vi "PathPlanning-int.vi"(0 "Map&Nodes":T1, 1 "error in (no error)":errorcluster) -> (2 "Path":i32[](array[numeric]), 3 "Coordinates":cluster{"X":dbl, "Y":dbl}[](array[cluster]), 4 "error out":errorcluster)   [LabVIEW 2009]
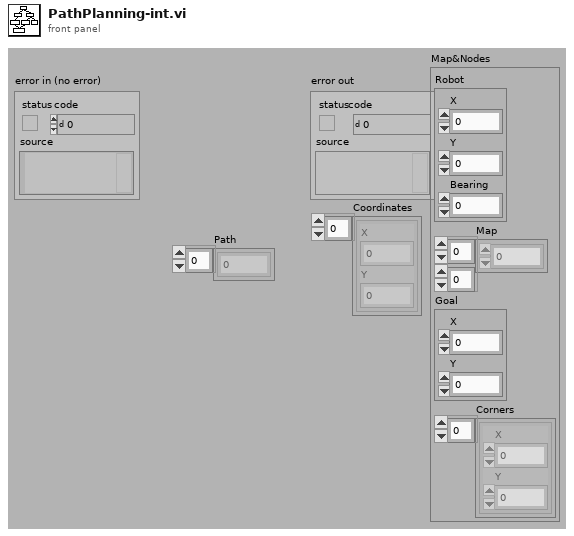
[diagram p1: front panel]
types:
  T1 = cluster{"Robot":cluster{"X":i16, "Y":i16, "Bearing":dbl}, "Map":i8[][], "Goal":cluster{"X":i16, "Y":i16}, "Corners":cluster{"X":i16, "Y":i16}[]}
  T2 = cluster{"From node":cluster{"X":i16, "Y":i16}, "Dest node":cluster{"X":i16, "Y":i16}, "Distance":dbl, "Dest node no":i32, "From node no":i32}[]
  T3 = cluster{"From node":cluster{"X":i16, "Y":i16}, "Dest node":cluster{"X":i16, "Y":i16}, "Distance":dbl, "Dest node no":i32, "From node no":i32}
  T4 = cluster{"From node":cluster{"X":dbl, "Y":dbl}, "Dest node":cluster{"X":dbl, "Y":dbl}, "Distance":dbl, "Dest node no":i32, "From node no":i32}
  T5 = cluster{"From node":cluster{"X":dbl, "Y":dbl}, "Dest node":cluster{"X":dbl, "Y":dbl}, "Distance":dbl, "Dest node no":i32, "From node no":i32}[]
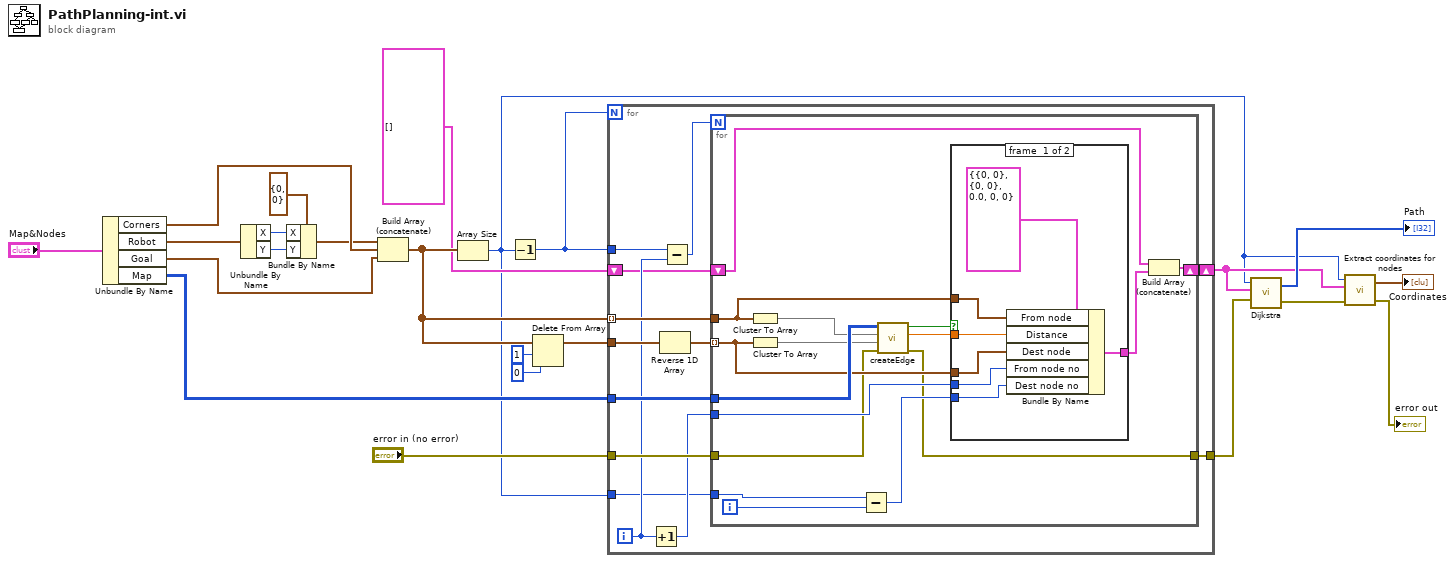
[diagram p0: block diagram]
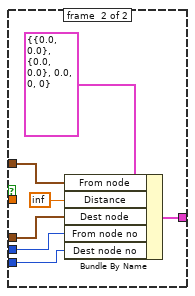
[diagram p2: hidden frame]
diagram:
  n1 = Unbundle By Name("Map&Nodes") -> ("Corners"=w15:cluster{"X":i16, "Y":i16}[], "Robot"=w19:cluster{"X":i16, "Y":i16, "Bearing":dbl}, "Goal"=w14:cluster{"X":i16, "Y":i16}, "Map"=w20:i8[][])
  n2 = Unbundle By Name(w19) -> ("X"=w18:i16, "Y"=w17:i16)
  n3 = Bundle By Name(cluster=cluster{"X":i16, "Y":i16} {"X"=0, "Y"=0} ("Robot 2"), "X"=w18, "Y"=w17) -> (w13:cluster{"X":i16, "Y":i16})
  n4 = Build Array (concatenate)(w13, w15, w14) -> (w12:cluster{"X":i16, "Y":i16}[])
  n5 = Array Size(array=w12) -> (size(s)=w2:i32)
  n6 = Decrement(x=w2) -> (x-1=w5:i32)
  n7 = Delete From Array(array=w12, length=1, index=0) -> (array with subset deleted=w21:cluster{"X":i16, "Y":i16}[])  [unwired: 1 out]
  n8 = for {
    N: w5 -> [_]
    tunnel: w12 -> [w35] mode=indexing
    tunnel: w21 -> [w36]
    tunnel: w20 -> [w34]
    tunnel: w5 -> [w32]
    tunnel: "error in (no error)" -> [w30]
    tunnel: [w29] -> w10
    shift-right: [w33] -> w4
    shift-left: T2 [] -> [w25]
    tunnel: w2 -> [w24]
    i -> [w28]
    n9 = Increment(x=w28) -> (x+1=w27:i32)
    n10 = Reverse 1D Array(array=w36) -> (reversed array=w26:cluster{"X":i16, "Y":i16}[])
    n11 = Subtract(x=w32, y=w28) -> (x-y=w31:i32)
    n12 = for {
      N: w31 -> [_]
      tunnel: w26 -> [w48] mode=indexing
      tunnel: w35 -> [w46]
      tunnel: w34 -> [w52]
      tunnel: w27 -> [w44]
      tunnel: w30 -> [w43]
      tunnel: [w42] -> w29
      shift-right: [w41] -> w33
      shift-left: w25 -> [w39]
      tunnel: w24 -> [w37]
      i -> [w38]
      n13 = Cluster To Array(cluster=w46) -> (array=w50:i16[])
      n14 = Cluster To Array(cluster=w48) -> (array=w49:i16[])
      n15 = Subtract(x=w37, y=w38) -> (x-y=w45:i32)
      n16 = call "createEdge.vi"("error in (no error)"=w43, "node 2"=w49, "node1"=w50, "Map"=w52) -> ("error out"=w42:errorcluster, "Distance"=w47:dbl, "FreePath"=w51:bool)  [unwired: 2 in]
      n17 = case shown="True" w51 {
        tunnel: w48 -> [w55 w63]
        tunnel: w47 -> [w58 _]
        tunnel: w46 -> [w59 w66]
        tunnel: [w56 w64] -> w40
        tunnel: w44 -> [w54 w62]
        tunnel: w45 -> [w53 w61]
        frame #0 {
          n18 = Bundle By Name(cluster=T3 {"From node"={"X"=0, "Y"=0}, "Dest node"={"X"=0, "Y"=0}, "Distance"=0.0, "Dest node no"=0, "From node no"=0}, "From node"=w59, "Distance"=w58, "Dest node"=w55, "From node no"=w54, "Dest node no"=w53) -> (w56:T3)
        }
        frame #1 {
          n19 = Bundle By Name(cluster=T4 {"From node"={"X"=0.0, "Y"=0.0}, "Dest node"={"X"=0.0, "Y"=0.0}, "Distance"=0.0, "Dest node no"=0, "From node no"=0}, "From node"=w66, "Distance"=inf, "Dest node"=w63, "From node no"=w62, "Dest node no"=w61) -> (w64:T4)
        }
      }
      n20 = Build Array (concatenate)(w39, w40) -> (w41:T5)
    }
  }
  n21 = call "Dijkstra.vi"("error in (no error)"=w10, "Edges"=w4, "Number of Nodes"=w2) -> ("error out"=w7:errorcluster, "Path"=→"Path":i32[])  [unwired: 1 in]
  n22 = call "Extract coordinates for nodes.vi"("error in (no error)"=w7, "Edges"=w4, "Number of Nodes"=w2) -> ("error out"=→"error out":errorcluster, "Coordinates"=→"Coordinates":cluster{"X":dbl, "Y":dbl}[])  [unwired: 1 in]
